vi "Write Key Value - Array (String).vi"(7 "Value":string[](array[string]), 8 "error in (no error)":errorcluster, 9 "key":string, 10 "section":string, 11 "file refnum in":T1) -> (0 "error out":errorcluster, 3 "file refnum out":T1)   [LabVIEW 2019, in "TSC File IO.lvlib"]
doc: "This VI will write a section/key configuration file of the type:\n<b>array of strings</b>\n\nInputs:\n-Path [path] - a path to the file\n-section [string] - the section string in the configuration file\n-key [string] - the key to be read in the configuration file\n-value [array of String] - the output data written\n-error in\n\nOutputs:\n-error out\n\n<b>Code Developed By:</b>\nDaniel Coons\nTechnology Service Corporation\n1983 S Liberty Drive\nBloomington, IN 47403\nwww.tsc.com\\atcs"
uses:
  TSC File IO.lvlib
  <vilib>/Utility/config.llb/NI_LVConfig.lvlib
  <vilib>/Utility/config.llb/Write Key (String).vi
  <vilib>/Utility/config.llb/Config Data RefNum.ctl
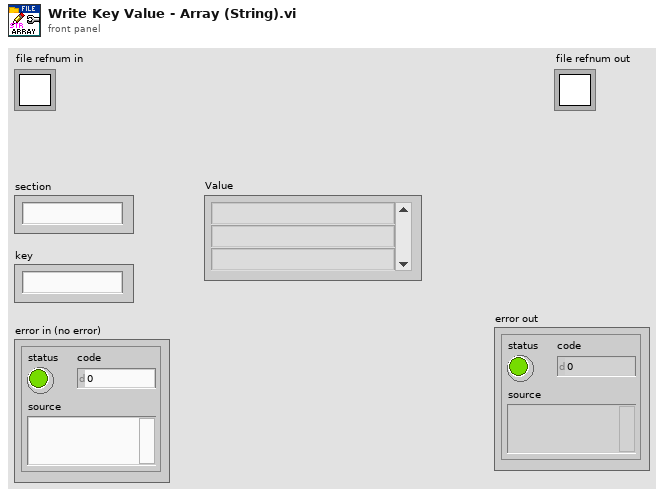
[diagram p1: front panel]
types:
  T1 = typedef "NI_LVConfig.lvlib/Config Data RefNum.ctl" = refnum<k1>
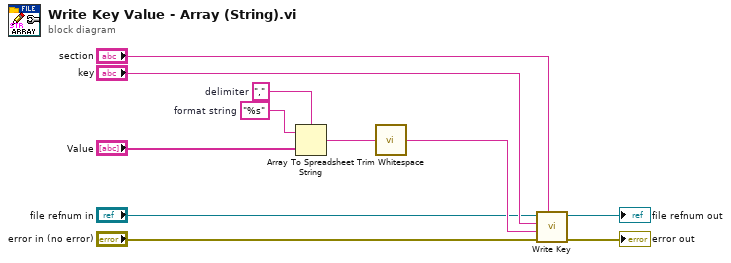
[diagram p0: block diagram]
diagram:
  w8 = "%s"  # format string
  w9 = ","  # delimiter
  n1 = Array To Spreadsheet String(delimiter (Tab)=w9, array="Value", 3:w8) -> (spreadsheet string=w6:string)
  n2 = call <vilib>:"Trim Whitespace.vi"("string"=w6) -> ("trimmed string"=w5:string)  [unwired: 1 in]
  n3 = call-poly <vilib>:"Write Key.vi"("section"="section", "error in (no error)"="error in (no error)", "value"=w5, "key"="key", "refnum"="file refnum in") -> ("error out"=→"error out":errorcluster, "refnum out"=→"file refnum out":T1)  [unwired: 4 in, 1 out]
